vi "robotAlign.vi"(9 "Target?":bool, 10 "Target Yaw":dbl, 11 "Numeric":dbl) -> (3 "output":dbl)   [LabVIEW 2023]
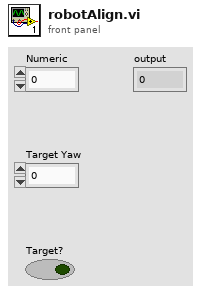
[diagram p1: front panel]
types:
  T1 = cluster{"proportional gain (Kp)":dbl, "integral time (Ki)":dbl, "derivative time (Kd)":dbl}
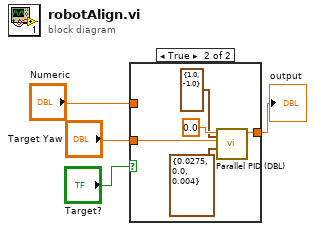
[diagram p0: block diagram]
diagram:
  n1 = case shown="True" "Target?" {
    tunnel: "Target Yaw" -> [_ w9]
    tunnel: [w5 w6] -> w1
    tunnel: "Numeric" -> [w5 _]
    frame False {
    }
    frame True {
      n2 = call <vilib>:"Parallel PID (DBL).vi"("output range"=cluster{"high":dbl, "low":dbl} {"high"=1.0, "low"=-1.0}, "PID gains"=T1 {"proportional gain (Kp)"=0.0275, "integral time (Ki)"=0.0, "derivative time (Kd)"=0.004}, "process variable"=w9, "setpoint"=0.0) -> ("output"=w6:dbl)  [unwired: 4 in, 3 out]
    }
  }
  "output" <- w1
